vi "autopilot.vi"() -> ()   [LabVIEW 2015]
uses:
  global.vi
  <vilib>/addons/control/pid/pid.llb/PID (DBL).vi
  <vilib>/addons/control/pid/NI_PID_pid.lvlib
  <vilib>/ptbypt/NI_PtbyPt.lvlib
panel:
  in  "Altitude":dbl
  in  "Target heading":dbl
  in  "Vertical speed":dbl
  in  "stop":bool
  in  "Airspeed knots":dbl
  in  "Pitch deg":dbl
  in  "Throttle control":bool
  in  "Pitch hold":T1(radio)
  in  "Roll hold":enum32{"OFF", "Roll hold", "Heading hold"}(radio)
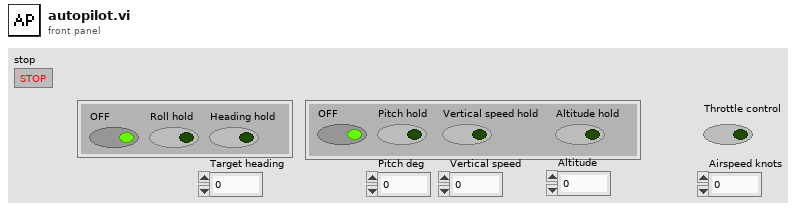
[diagram p1: front panel]
types:
  T1 = enum32{"OFF", "Pitch hold", "Vertical speed hold", "Altitude hold"}
  T2 = typedef "Window Refnum" = refnum<k1>
  T3 = cluster{"Airspeed":dbl, "Altitude":dbl, "Vertical Speed":dbl, "Pitch":dbl, "Roll":dbl, "Heading":dbl, "Turn Indicator":dbl, "Latitude":dbl, "Longitude":dbl}
  T4 = cluster{"setpoint":dbl, "setpoint":dbl, "setpoint":dbl}
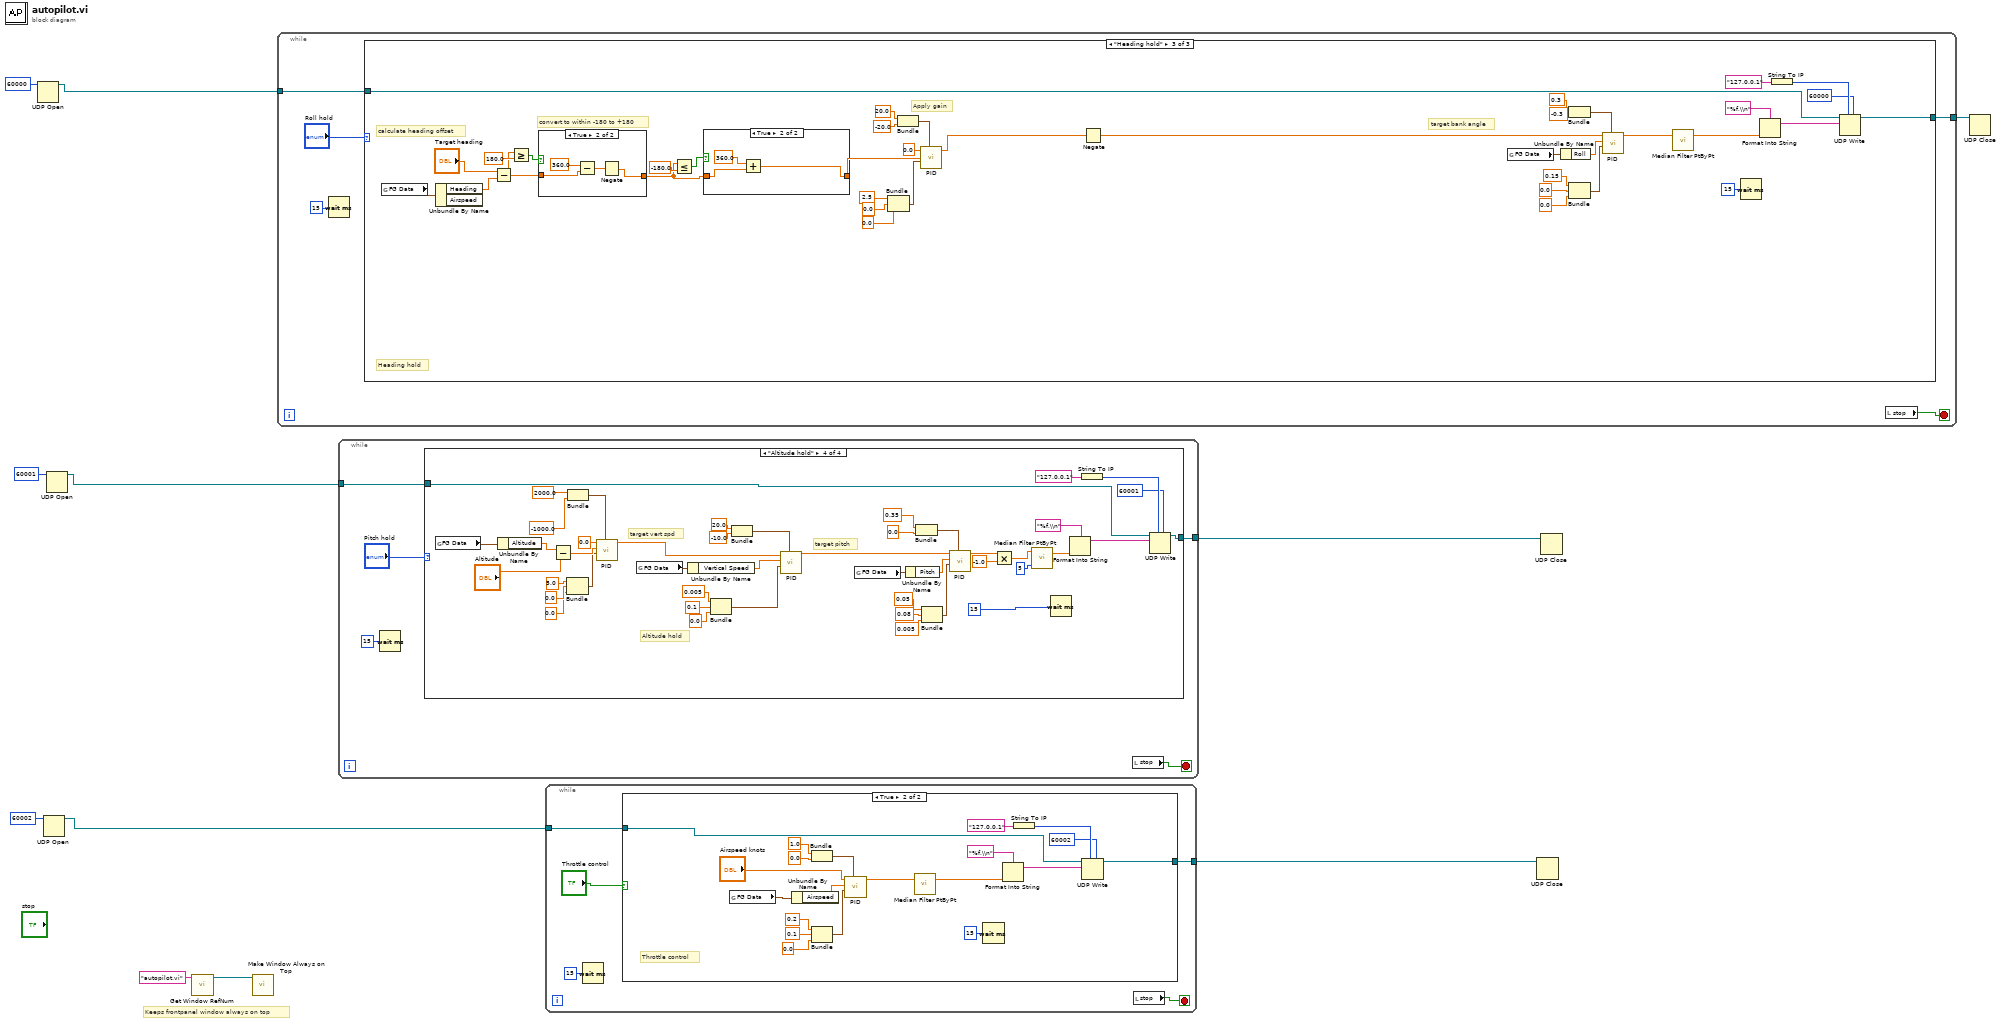
[diagram p0: block diagram]
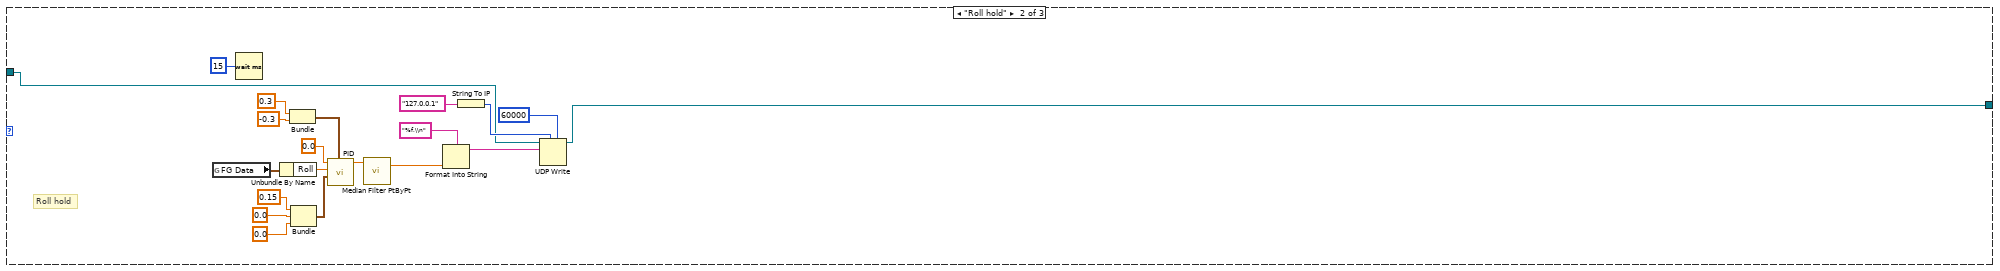
[diagram p3: hidden frame]
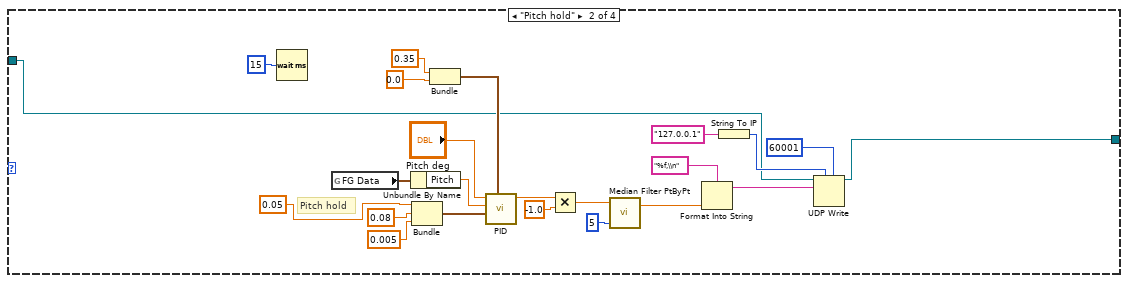
[diagram p7: hidden frame]
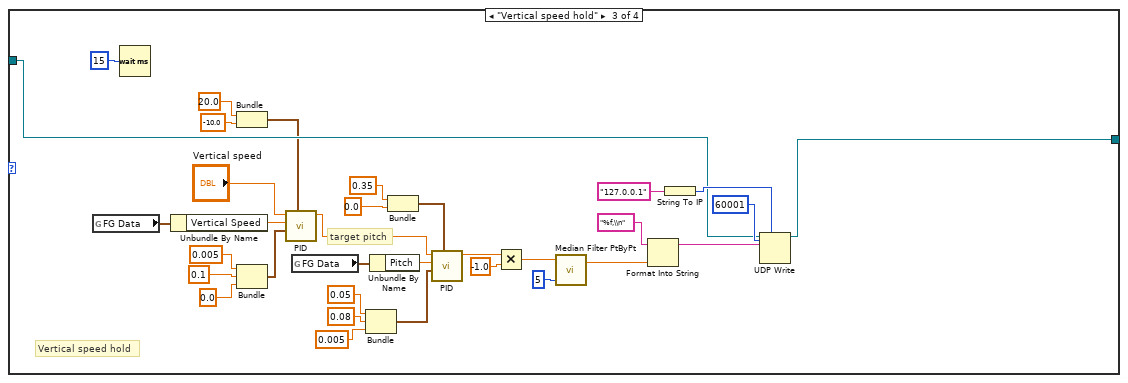
[diagram p8: hidden frame]
diagram:
  # "Keeps frontpanel window always on top"
  n1 = UDP Open(11:u16 60000 ("port")) -> (port=w4:refnum<k16>)  [unwired: 4 in, 2 out]
  n2 = UDP Open(11:u16 60002 ("port")) -> (port=w7:refnum<k16>)  [unwired: 4 in, 2 out]
  n3 = UDP Open(11:u16 60001 ("port")) -> (port=w10:refnum<k16>)  [unwired: 4 in, 2 out]
  n4 = call "Get Window RefNum.vi"("window name (\"\")"="autopilot.vi" ("window name (\"\")")) -> ("window refnum (NaWR)"=w1:T2)  [unwired: 7 in, 1 out]
  n5 = call "Make Window Always on Top.vi"("window refnum (NaWR)"=w1) -> ()  [unwired: 5 in, 2 out]
  n6 = while {
    tunnel: w4 -> [w14]
    tunnel: [w13] -> w3
    stop <- w15 stop-if-true
    n7 = Wait (ms)(milliseconds to wait=u32 15) -> ()  [unwired: 1 out]
    n8 = case shown="\"Heading hold\"" "Roll hold" {
      tunnel: w14 -> [w17 w19 w59]
      tunnel: [w17 w18 w58] -> w13
      frame "OFF", Default {
      }
      frame "Roll hold" {
        # "Roll hold"
        n9 = global read "global.vi" "FG Data"() -> (w28:T3)
        n10 = Wait (ms)(milliseconds to wait=u32 15) -> ()  [unwired: 1 out]
        n11 = Unbundle By Name(w28) -> ("Roll"=w37:dbl)
        n12 = Bundle(0.3, -0.3) -> (w31:cluster{dbl, dbl})  [unwired: 1 in]
        n13 = Bundle(0.15, 0.0, 0.0) -> (w34:cluster{dbl, dbl, dbl})  [unwired: 1 in]
        n14 = call-poly <vilib>:"PID.vi"("output range"=w31, "PID gains"=w34, "process variable"=w37, "setpoint"=0.0) -> ("output"=w22:dbl)  [unwired: 6 in, 1 out]
        n15 = call <vilib>:"Median Filter PtByPt.vi"("x"=w22) -> ("Filtered x"=w21:dbl)  [unwired: 3 in, 1 out]
        n16 = Format Into String(format string="%f,\\n", w21) -> (resulting string=w23:string)  [unwired: 2 in, 1 out]
        n17 = String To IP(1:"127.0.0.1" ("name")) -> (0:w26:u32)
        n18 = UDP Write(address=w26, port or service name=u16 60000, connection ID=w19, data in=w23) -> (3:w18:refnum<k16>)  [unwired: 2 in, 1 out]
      }
      frame "Heading hold" {
        # "convert to within -180 to +180"
        # "target bank angle"
        # "Apply gain"
        # "calculate heading offset"
        # "Heading hold"
        n19 = global read "global.vi" "FG Data"() -> (w57:T3)
        n20 = Unbundle By Name(w57) -> ("Heading"=w55:dbl)  [unwired: 1 out]
        n21 = Subtract(x="Target heading", y=w55) -> (x-y=w52:dbl)
        n22 = Greater Or Equal?(x=w52, y=180.0) -> (x >= y?=w53:bool)
        n23 = case shown="True" w53 {
          tunnel: w52 -> [w81 w85]
          tunnel: [w81 w82] -> w49
          frame False {
          }
          frame True {
            n24 = Subtract(x=360.0, y=w85) -> (x-y=w83:dbl)
            n25 = Negate(x=w83) -> (-x=w82:dbl)
          }
        }
        n26 = Less Or Equal?(x=w49, y=-180.0) -> (x <= y?=w50:bool)
        n27 = case shown="True" w50 {
          tunnel: w49 -> [w77 w80]
          tunnel: [w77 w78] -> w40
          frame False {
          }
          frame True {
            n28 = Add(x=360.0, y=w80) -> (x+y=w78:dbl)
          }
        }
        n29 = Bundle("x"=2.5, "x"=0.0, "x"=0.0) -> (w48:cluster{"x":dbl, "x":dbl, "x":dbl})  [unwired: 1 in]
        n30 = Bundle("x"=20.0, "x"=-20.0) -> (w42:cluster{"x":dbl, "x":dbl})  [unwired: 1 in]
        n31 = call-poly <vilib>:"PID.vi"("output range"=w42, "PID gains"=w48, "process variable"=w40, "setpoint"=0.0) -> ("output"=w39:dbl)  [unwired: 6 in, 1 out]
        n32 = Negate(x=w39) -> (-x=w38:dbl)
        n33 = global read "global.vi" "FG Data"() -> (w68:T3)
        n34 = Unbundle By Name(w68) -> ("Roll"=w76:dbl)
        n35 = Bundle(0.3, -0.3) -> (w71:cluster{dbl, dbl})  [unwired: 1 in]
        n36 = Bundle(0.15, 0.0, 0.0) -> (w74:cluster{dbl, dbl, dbl})  [unwired: 1 in]
        n37 = call-poly <vilib>:"PID.vi"("output range"=w71, "PID gains"=w74, "process variable"=w76, "setpoint"=w38) -> ("output"=w62:dbl)  [unwired: 6 in, 1 out]
        n38 = call <vilib>:"Median Filter PtByPt.vi"("x"=w62) -> ("Filtered x"=w61:dbl)  [unwired: 3 in, 1 out]
        n39 = Wait (ms)(milliseconds to wait=u32 15) -> ()  [unwired: 1 out]
        n40 = Format Into String(format string="%f,\\n", w61) -> (resulting string=w63:string)  [unwired: 2 in, 1 out]
        n41 = String To IP(1:"127.0.0.1" ("name")) -> (0:w66:u32)
        n42 = UDP Write(address=w66, port or service name=u16 60000, connection ID=w59, data in=w63) -> (3:w58:refnum<k16>)  [unwired: 2 in, 1 out]
      }
    }
    n43 = local read "stop"() -> (w15:bool)
  }
  n44 = while {
    tunnel: w10 -> [w88]
    tunnel: [w87] -> w9
    stop <- w89 stop-if-true
    n45 = Wait (ms)(milliseconds to wait=u32 15) -> ()  [unwired: 1 out]
    n46 = case shown="\"Altitude hold\"" "Pitch hold" {
      tunnel: w88 -> [w91 w94 w128 w173]
      tunnel: [w91 w93 w127 w172] -> w87
      frame "OFF", Default {
      }
      frame "Pitch hold" {
        # "Pitch hold"
        n47 = Wait (ms)(milliseconds to wait=u32 15) -> ()  [unwired: 1 out]
        n48 = global read "global.vi" "FG Data"() -> (w106:T3)
        n49 = Unbundle By Name(w106) -> ("Pitch"=w114:dbl)
        n50 = Bundle(0.05, 0.08, 0.005) -> (w112:cluster{dbl, dbl, dbl})  [unwired: 1 in]
        n51 = Bundle(0.35, 0.0) -> (w109:cluster{dbl, dbl})  [unwired: 1 in]
        n52 = call-poly <vilib>:"PID.vi"("output range"=w109, "PID gains"=w112, "process variable"=w114, "setpoint"="Pitch deg") -> ("output"=w97:dbl)  [unwired: 6 in, 1 out]
        n53 = Multiply(x=w97, y=-1.0) -> (x*y=w98:dbl)
        n54 = call <vilib>:"Median Filter PtByPt.vi"("rank"=5, "x"=w98) -> ("Filtered x"=w99:dbl)  [unwired: 2 in, 1 out]
        n55 = Format Into String(format string="%f,\\n", w99) -> (resulting string=w101:string)  [unwired: 2 in, 1 out]
        n56 = String To IP(1:"127.0.0.1" ("name")) -> (0:w104:u32)
        n57 = UDP Write(address=w104, port or service name=u16 60001, connection ID=w94, data in=w101) -> (3:w93:refnum<k16>)  [unwired: 2 in, 1 out]
      }
      frame "Vertical speed hold" {
        # "target pitch"
        # "Vertical speed hold"
        n58 = global read "global.vi" "FG Data"() -> (w119:T3)
        n59 = Wait (ms)(milliseconds to wait=u32 15) -> ()  [unwired: 1 out]
        n60 = Unbundle By Name(w119) -> ("Vertical Speed"=w118:dbl)
        n61 = Bundle(20.0, -10.0) -> (w126:cluster{dbl, dbl})  [unwired: 1 in]
        n62 = Bundle(0.005, 0.1, 0.0) -> (w117:cluster{dbl, dbl, dbl})  [unwired: 1 in]
        n63 = call-poly <vilib>:"PID.vi"("output range"=w126, "PID gains"=w117, "process variable"=w118, "setpoint"="Vertical speed") -> ("output"=w115:dbl)  [unwired: 6 in, 1 out]
        n64 = global read "global.vi" "FG Data"() -> (w139:T3)
        n65 = Bundle(0.05, 0.08, 0.005) -> (w145:cluster{dbl, dbl, dbl})  [unwired: 1 in]
        n66 = Unbundle By Name(w139) -> ("Pitch"=w147:dbl)
        n67 = Bundle(0.35, 0.0) -> (w142:cluster{dbl, dbl})  [unwired: 1 in]
        n68 = call-poly <vilib>:"PID.vi"("output range"=w142, "PID gains"=w145, "process variable"=w147, "setpoint"=w115) -> ("output"=w130:dbl)  [unwired: 6 in, 1 out]
        n69 = Multiply(x=w130, y=-1.0) -> (x*y=w131:dbl)
        n70 = call <vilib>:"Median Filter PtByPt.vi"("rank"=5, "x"=w131) -> ("Filtered x"=w132:dbl)  [unwired: 2 in, 1 out]
        n71 = Format Into String(format string="%f,\\n", w132) -> (resulting string=w134:string)  [unwired: 2 in, 1 out]
        n72 = String To IP(1:"127.0.0.1" ("name")) -> (0:w137:u32)
        n73 = UDP Write(address=w137, port or service name=u16 60001, connection ID=w128, data in=w134) -> (3:w127:refnum<k16>)  [unwired: 2 in, 1 out]
      }
      frame "Altitude hold" {
        # "target vert spd"
        # "target pitch"
        # "Altitude hold"
        n74 = global read "global.vi" "FG Data"() -> (w161:T3)
        n75 = Unbundle By Name(w161) -> ("Altitude"=w151:dbl)
        n76 = Subtract(x=w151, y="Altitude") -> (x-y=w160:dbl)
        n77 = Bundle("setpoint"=5.0, "setpoint"=0.0, "setpoint"=0.0) -> (w157:T4)  [unwired: 1 in]
        n78 = Bundle("setpoint"=2000.0, "setpoint"=-1000.0) -> (w158:cluster{"setpoint":dbl, "setpoint":dbl})  [unwired: 1 in]
        n79 = call-poly <vilib>:"PID.vi"("output range"=w158, "PID gains"=w157, "process variable"=w160, "setpoint"=0.0) -> ("output"=w148:dbl)  [unwired: 6 in, 1 out]
        n80 = global read "global.vi" "FG Data"() -> (w165:T3)
        n81 = Unbundle By Name(w165) -> ("Vertical Speed"=w164:dbl)
        n82 = Bundle(0.005, 0.1, 0.0) -> (w163:cluster{dbl, dbl, dbl})  [unwired: 1 in]
        n83 = Bundle(20.0, -10.0) -> (w171:cluster{dbl, dbl})  [unwired: 1 in]
        n84 = call-poly <vilib>:"PID.vi"("output range"=w171, "PID gains"=w163, "process variable"=w164, "setpoint"=w148) -> ("output"=w149:dbl)  [unwired: 6 in, 1 out]
        n85 = global read "global.vi" "FG Data"() -> (w184:T3)
        n86 = Unbundle By Name(w184) -> ("Pitch"=w192:dbl)
        n87 = Bundle(0.35, 0.0) -> (w187:cluster{dbl, dbl})  [unwired: 1 in]
        n88 = Bundle(0.05, 0.08, 0.005) -> (w190:cluster{dbl, dbl, dbl})  [unwired: 1 in]
        n89 = call-poly <vilib>:"PID.vi"("output range"=w187, "PID gains"=w190, "process variable"=w192, "setpoint"=w149) -> ("output"=w175:dbl)  [unwired: 6 in, 1 out]
        n90 = Multiply(x=w175, y=-1.0) -> (x*y=w176:dbl)
        n91 = call <vilib>:"Median Filter PtByPt.vi"("rank"=5, "x"=w176) -> ("Filtered x"=w177:dbl)  [unwired: 2 in, 1 out]
        n92 = Wait (ms)(milliseconds to wait=u32 15) -> ()  [unwired: 1 out]
        n93 = Format Into String(format string="%f,\\n", w177) -> (resulting string=w179:string)  [unwired: 2 in, 1 out]
        n94 = String To IP(1:"127.0.0.1" ("name")) -> (0:w182:u32)
        n95 = UDP Write(address=w182, port or service name=u16 60001, connection ID=w173, data in=w179) -> (3:w172:refnum<k16>)  [unwired: 2 in, 1 out]
      }
    }
    n96 = local read "stop"() -> (w89:bool)
  }
  n97 = while {
    tunnel: w7 -> [w195]
    tunnel: [w194] -> w6
    stop <- w196 stop-if-true
    n98 = Wait (ms)(milliseconds to wait=u32 15) -> ()  [unwired: 1 out]
    n99 = case shown="True" "Throttle control" {
      tunnel: w195 -> [w198 w200]
      tunnel: [w198 w199] -> w194
      frame False {
      }
      frame True {
        # "Throttle control"
        n100 = global read "global.vi" "FG Data"() -> (w210:T3)
        n101 = Unbundle By Name(w210) -> ("Airspeed"=w218:dbl)
        n102 = Bundle(1.0, 0.0) -> (w213:cluster{dbl, dbl})  [unwired: 1 in]
        n103 = Bundle(0.2, 0.1, 0.0) -> (w216:cluster{dbl, dbl, dbl})  [unwired: 1 in]
        n104 = call-poly <vilib>:"PID.vi"("output range"=w213, "PID gains"=w216, "process variable"=w218, "setpoint"="Airspeed knots") -> ("output"=w204:dbl)  [unwired: 6 in, 1 out]
        n105 = call <vilib>:"Median Filter PtByPt.vi"("x"=w204) -> ("Filtered x"=w203:dbl)  [unwired: 3 in, 1 out]
        n106 = Wait (ms)(milliseconds to wait=u32 15) -> ()  [unwired: 1 out]
        n107 = Format Into String(format string="%f,\\n", w203) -> (resulting string=w205:string)  [unwired: 2 in, 1 out]
        n108 = String To IP(1:"127.0.0.1" ("name")) -> (0:w208:u32)
        n109 = UDP Write(address=w208, port or service name=u16 60002, connection ID=w200, data in=w205) -> (3:w199:refnum<k16>)  [unwired: 2 in, 1 out]
      }
    }
    n110 = local read "stop"() -> (w196:bool)
  }
  n111 = UDP Close(connection ID=w6) -> ()  [unwired: 1 in, 2 out]
  n112 = UDP Close(connection ID=w9) -> ()  [unwired: 1 in, 2 out]
  n113 = UDP Close(connection ID=w3) -> ()  [unwired: 1 in, 2 out]
